vi "SetupGraph.vi"(0 "trigger level":dbl, 1 "Scaling Factor":dbl, 2 "input capture cluster":T2, 3 "Minimum Y":dbl) -> (4 "current only plot":T1, 6 "mean":dbl format="%0.2f", 7 "output plot":cluster{i32, "xIncrement":dbl, dbl[][]}, 8 "standard deviation":dbl format="%0.2f", 9 "variance":dbl format="%0.2f")   [LabVIEW 2012]
uses:
  <vilib>/Analysis/NI_AALBase.lvlib
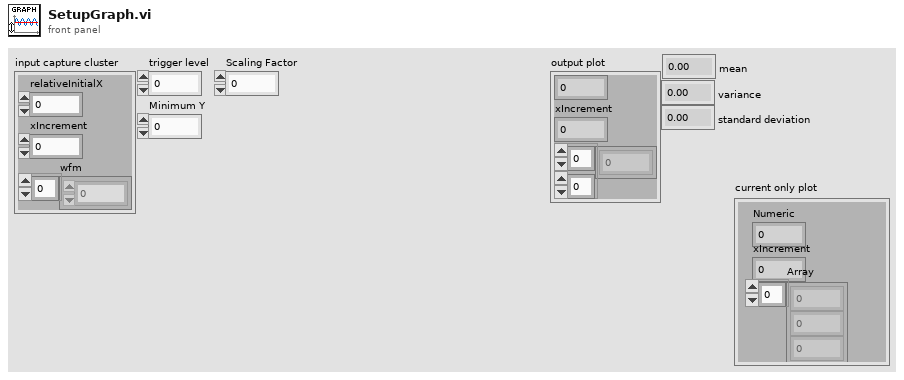
[diagram p1: front panel]
types:
  T1 = cluster{"Numeric":i32, "xIncrement":dbl, "Array":dbl[]}
  T2 = cluster{"relativeInitialX":dbl, "xIncrement":dbl, "wfm":dbl[]}
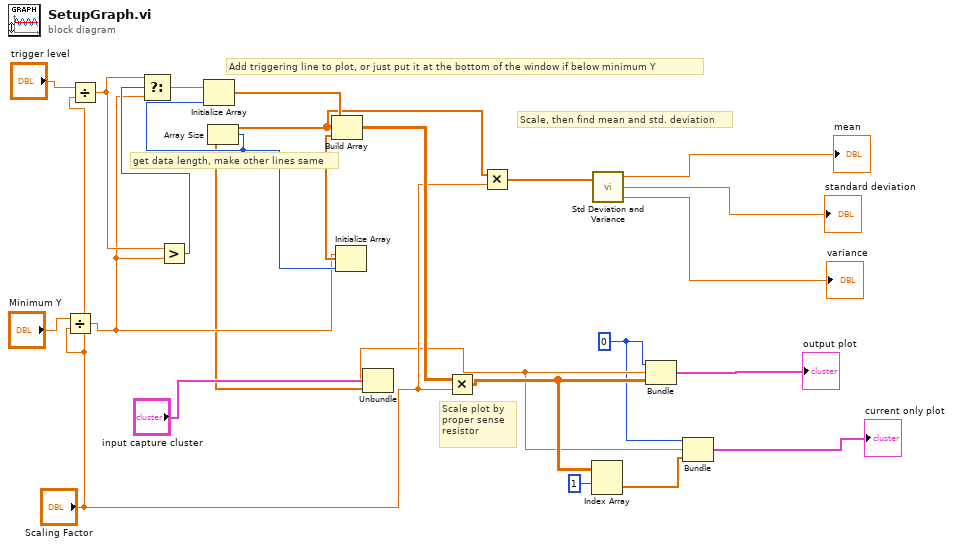
[diagram p0: block diagram]
diagram:
  w3 = 0
  # "Scale, then find mean and std. deviation"
  # "get data length, make other lines same"
  # "Add triggering line to plot, or just put it at the bottom of the window if below minimum Y"
  # "Scale plot by proper sense resistor"
  n1 = Divide(x="Minimum Y", y="Scaling Factor") -> (x/y=w13:dbl)
  n2 = Divide(x="trigger level", y="Scaling Factor") -> (x/y=w15:dbl)
  n3 = Greater?(x=w15, y=w13) -> (0:w18:bool)
  n4 = Select(t=w15, s=w18, f=w13) -> (s? t:f=w17:dbl)
  n5 = Unbundle("input capture cluster") -> ("xIncrement"=w4:dbl, "wfm"=w10:dbl[])  [unwired: 1 out]
  n6 = Array Size(array=w10) -> (size(s)=w21:i32)
  n7 = Initialize Array(w17, w21) -> (w23:dbl[])
  n8 = Initialize Array(w13, w21) -> (w22:dbl[])
  n9 = Build Array(w23, w10, w22) -> (w24:dbl[][])
  n10 = Multiply(x=w24, y="Scaling Factor") -> (x*y=w6:dbl[][])
  n11 = Multiply(x=w10, y="Scaling Factor") -> (x*y=w11:dbl[])
  n12 = Index Array(array=w6, index (row)=1 ("index(row)")) -> (element=w2:dbl[])  [unwired: 1 in]
  n13 = call <vilib>:"Std Deviation and Variance.vi"("X"=w11) -> ("mean"=→"mean":dbl, "standard deviation"=→"standard deviation":dbl, "variance"=→"variance":dbl)  [unwired: 1 in]
  n14 = Bundle(w3, "xIncrement"=w4, w6) -> (→"output plot":cluster{i32, "xIncrement":dbl, dbl[][]})  [unwired: 1 in]
  n15 = Bundle(w3, "xIncrement"=w4, w2) -> (→"current only plot":cluster{i32, "xIncrement":dbl, dbl[]})  [unwired: 1 in]
